vi "SaveReport.vi"(8 "error in (no error)":errorcluster, 9 "Done":bool, 10 "TestResultInformation":T1, 11 "LocalReport in":refnum<class "LocalReport.lvclass">) -> (0 "error out":errorcluster, 3 "LocalReport out":refnum<class "LocalReport.lvclass">)   [LabVIEW 2019, in "LocalReport.lvlib" / "LocalReport.lvclass"]
uses:
  LocalReport.lvclass
  C:/Program Files (x86)/National Instruments/LabVIEW 2019/vi.lib/NI/Event Source Actor/Event Source/Event Source/Event Source.lvclass
  LocalReport.lvclass/LocalReport.ctl
  TestReport.lvclass
  C:/Program Files (x86)/National Instruments/LabVIEW 2019/vi.lib/NI/Event Source Actor/Event Source/Event/Event.lvclass
  <vilib>/NI/Event Source Actor/Event Source/Event/Event.lvclass/Event.ctl
  <vilib>/Utility/file.llb/Write Delimited Spreadsheet (string).vi
  <vilib>/NI/Event Source Actor/Event Source/Event/Event.lvclass
  <vilib>/NI/Event Source Actor/Event Source/Event Source/Event Source.lvclass
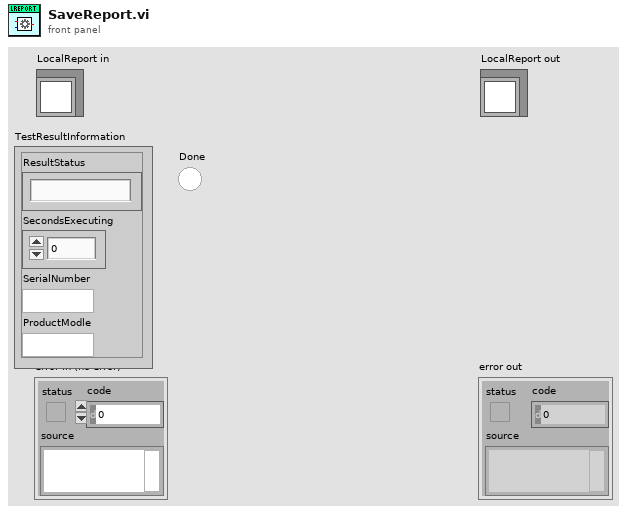
[diagram p1: front panel]
types:
  T1 = cluster{"ResultStatus":string, "SecondsExecuting":dbl, "SerialNumber":string, "ProductModle":string}
  T2 = cluster{"TestResultData":string[][], "SerialNumber":string}[]
  T3 = cluster{"TestResultData":string[][], "SerialNumber":string}
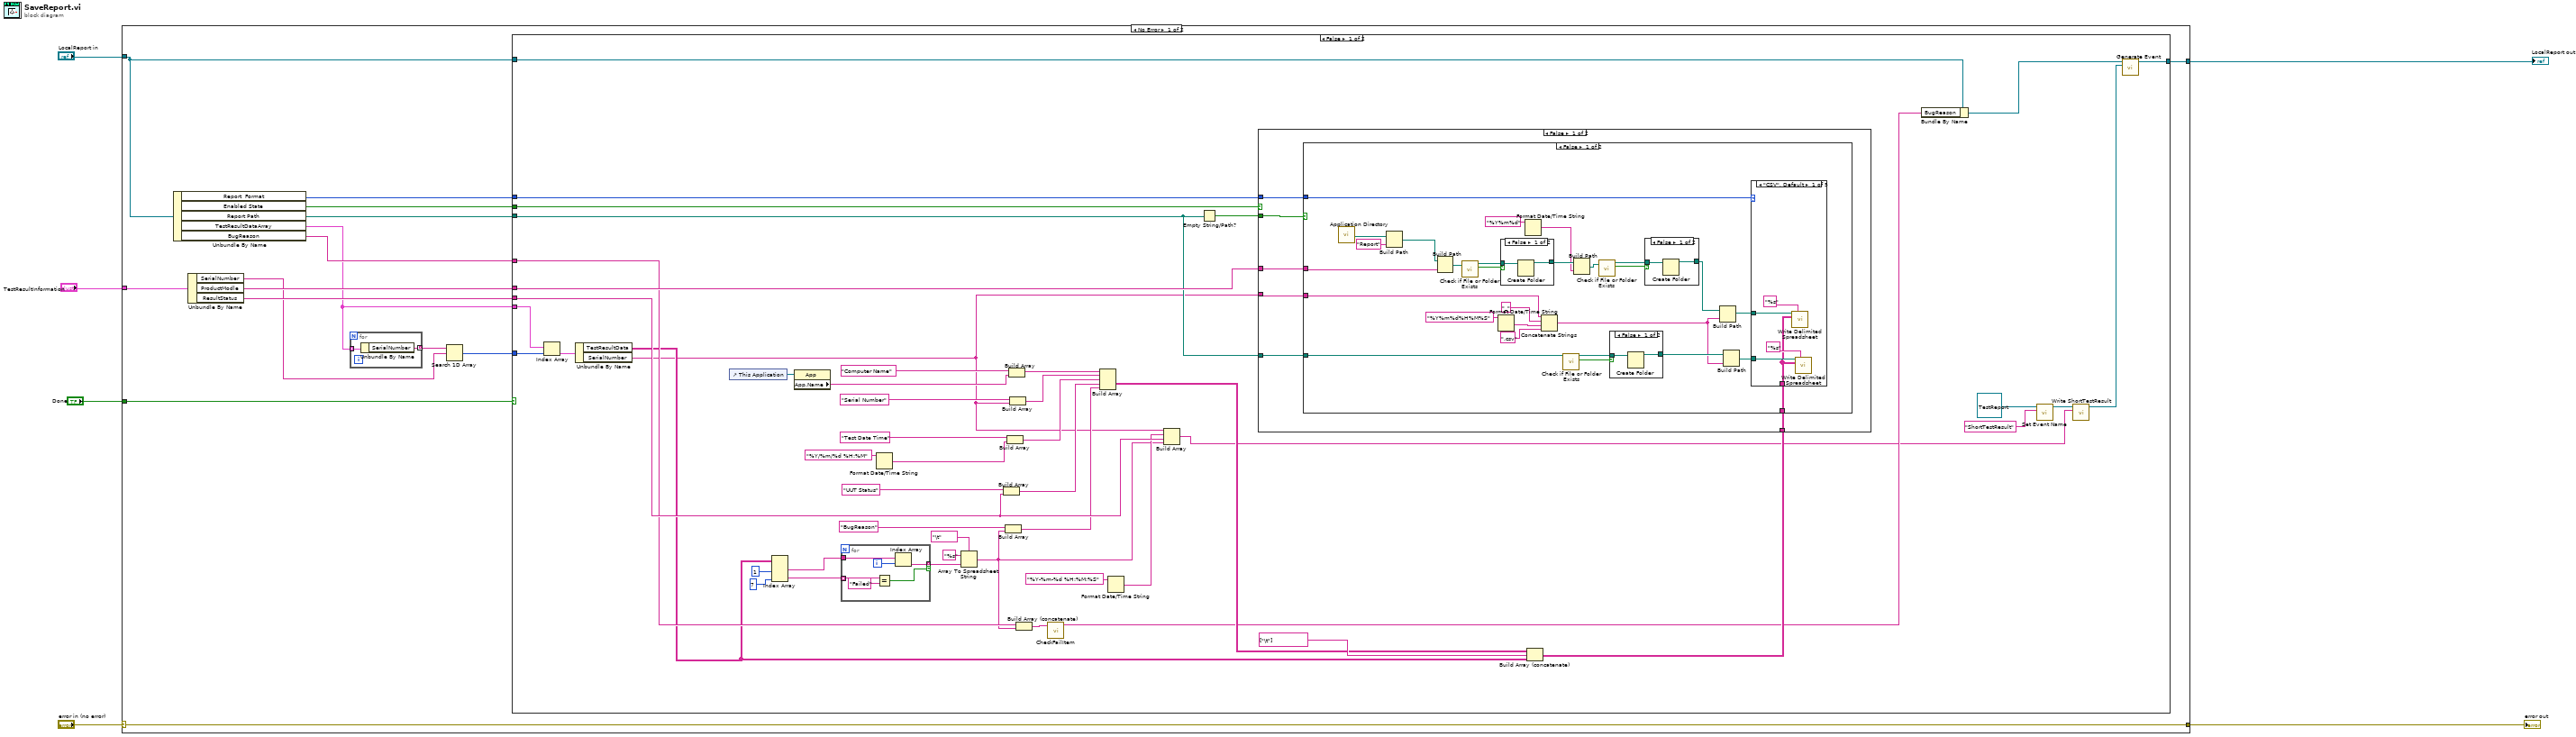
[diagram p0: block diagram]
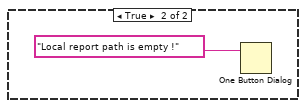
[diagram p9: hidden frame]
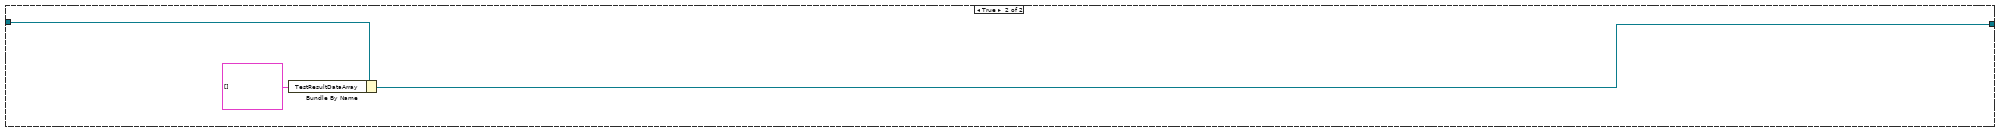
[diagram p11: hidden frame]
diagram:
  n1 = case shown="No Error" "error in (no error)" {
    selector: "error in (no error)" -> [w21 w132]
    tunnel: [w21 w132] -> w5
    tunnel: [w12 w131] -> w3
    tunnel: "LocalReport in" -> [w13 w131]
    tunnel: "TestResultInformation" -> [w20 _]
    tunnel: "Done" -> [w7 _]
    frame No Error {
      n2 = Unbundle By Name(w13) -> ("Report  Format"=w15:enum16{"CSV", "XML", "PDF", "Excel", "TXT"}, "Enabled State"=w16:bool, "Report Path"=w17:path, "TestResultDataArray"=w11:T2, "BugReason"=w14:string[])
      n3 = Unbundle By Name(w20) -> ("SerialNumber"=w9:string, "ProductModle"=w18:string, "ResultStatus"=w19:string)
      n4 = for {
        tunnel: w11 -> [w130] mode=indexing
        tunnel: [w129] -> w10 mode=indexing
        n5 = Unbundle By Name(w130) -> ("SerialNumber"=w129:string)
      }
      n6 = Search 1D Array(1D array=w10, element=w9) -> (index of element=w8:i32)  [unwired: 1 in]
      n7 = case shown="False" w7 {
        tunnel: w19 -> [w70 _]
        tunnel: w18 -> [w69 _]
        tunnel: w17 -> [w68 _]
        tunnel: w16 -> [w67 _]
        tunnel: w15 -> [w66 _]
        tunnel: w14 -> [w65 _]
        tunnel: w13 -> [w64 w128]
        tunnel: [w26 w126] -> w12
        tunnel: w11 -> [w23 _]
        tunnel: w8 -> [w22 _]
        frame False {
          n8 = Index Array(array=w23, index=w22) -> (element=w27:T3)
          n9 = Unbundle By Name(w27) -> ("TestResultData"=w28:string[][], "SerialNumber"=w24:string)
          n10 = control-ref of="This Application"() -> (w41:refnum<vi>)
          n11 = Index Array(array=w28, index (col) #1=1 ("disabled index (col)"), index (col) #2=7 ("disabled index (col)")) -> (element #1=w51:string[], element #2=w53:string[])  [unwired: 2 in]
          n12 = property class="App"(reference=w41) -> ("App.Name"=w40:string)  [unwired: 1 in, 2 out]
          n13 = for {
            tunnel: w53 -> [w125] mode=indexing
            tunnel: [w120] -> w50 mode=indexing if=w123
            tunnel: w51 -> [w121]
            i -> [w122]
            n14 = Equal?(x=w125, y="Failed") -> (x = y?=w123:bool)
            n15 = Index Array(array=w121, index=w122) -> (element=w120:string)
          }
          n16 = Format Date/Time String(time format string (%c)="%Y/%m/%d %H:%M") -> (date/time string=w43:string)  [unwired: 2 in]
          n17 = Array To Spreadsheet String(delimiter (Tab)="\t", array=w50, 3:"%s" ("format string")) -> (spreadsheet string=w25:string)
          n18 = Build Array("UUT Status", w70) -> (w56:string[])
          n19 = Build Array("BugReason", w25) -> (w47:string[])
          n20 = Build Array("Test Date Time", w43) -> (w57:string[])
          n21 = Build Array("Computer Name", w40) -> (w59:string[])
          n22 = Build Array("Serial Number", w24) -> (w58:string[])
          n23 = Build Array (concatenate)(w65, w25) -> (w38:string[])
          n24 = call "CheckFailItem.vi"("in"=w38) -> ("out"=w37:string[])  [unwired: 10 in]
          n25 = Build Array(w59, w58, w57, w56, w47) -> (w45:string[][])
          n26 = Format Date/Time String(time format string (%c)="%Y-%m-%d %H:%M:%S") -> (date/time string=w29:string)  [unwired: 2 in]
          n27 = Build Array(w24, w29, w70, w25) -> (w31:string[])
          n28 = Empty String/Path?(string/path=w68) -> (empty?=w39:bool)
          n29 = Build Array (concatenate)(w45, string[] ["\t"], w28) -> (w42:string[][])
          n30 = case shown="False" w67 {
            tunnel: w42 -> [w76 _]
            tunnel: w69 -> [w75 _]
            tunnel: w68 -> [w74 _]
            tunnel: w24 -> [w73 _]
            tunnel: w39 -> [w72 _]
            tunnel: w66 -> [w71 _]
            frame False {
              n31 = case shown="False" w72 {
                tunnel: w76 -> [w92 _]
                tunnel: w75 -> [w88 _]
                tunnel: w74 -> [w87 _]
                tunnel: w73 -> [w81 _]
                tunnel: w71 -> [w80 _]
                frame False {
                  n32 = call <vilib>:"Application Directory.vi"() -> ("Application Directory"=w79:path)
                  n33 = Build Path(base path=w79, name or relative path="Report") -> (appended path=w78:path)
                  n34 = Build Path(base path=w78, name or relative path=w88) -> (appended path=w103:path)
                  n35 = call <vilib>:"Check if File or Folder Exists.vi"("path"=w103) -> ("file or folder exists?"=w102:bool, "dup path"=w101:path)  [unwired: 8 in, 1 out]
                  n36 = Format Date/Time String(time format string (%c)="%Y%m%d%H%M%S") -> (date/time string=w86:string)  [unwired: 2 in]
                  n37 = case shown="False" w102 {
                    tunnel: w101 -> [w117 w118]
                    tunnel: [w116 w118] -> w100
                    frame False {
                      n38 = Create Folder(path (use dialog)=w117) -> (created path=w116:path)  [unwired: 2 in, 2 out]
                    }
                    frame True {
                    }
                  }
                  n39 = Format Date/Time String(time format string (%c)="%Y%m%d") -> (date/time string=w98:string)  [unwired: 2 in]
                  n40 = Concatenate Strings(w81, "_" ("string"), w86, ".csv" ("name or relative path")) -> (w82:string)
                  n41 = call <vilib>:"Check if File or Folder Exists.vi"("path"=w87) -> ("file or folder exists?"=w90:bool, "dup path"=w91:path)  [unwired: 8 in, 1 out]
                  n42 = Build Path(base path=w100, name or relative path=w98) -> (appended path=w95:path)
                  n43 = call <vilib>:"Check if File or Folder Exists.vi"("path"=w95) -> ("file or folder exists?"=w96:bool, "dup path"=w97:path)  [unwired: 8 in, 1 out]
                  n44 = case shown="False" w90 {
                    tunnel: w91 -> [w111 w112]
                    tunnel: [w110 w112] -> w89
                    frame False {
                      n45 = Create Folder(path (use dialog)=w111) -> (created path=w110:path)  [unwired: 2 in, 2 out]
                    }
                    frame True {
                    }
                  }
                  n46 = case shown="False" w96 {
                    tunnel: w97 -> [w114 w115]
                    tunnel: [w113 w115] -> w94
                    frame False {
                      n47 = Create Folder(path (use dialog)=w114) -> (created path=w113:path)  [unwired: 2 in, 2 out]
                    }
                    frame True {
                    }
                  }
                  n48 = Build Path(base path=w94, name or relative path=w82) -> (appended path=w104:path)
                  n49 = Build Path(base path=w89, name or relative path=w82) -> (appended path=w93:path)
                  n50 = case shown="\"CSV\", Default" w80 {
                    tunnel: w104 -> [w109 _ _ _ _]
                    tunnel: w93 -> [w106 _ _ _ _]
                    tunnel: w92 -> [w105 _ _ _ _]
                    frame "CSV", Default {
                      n51 = call-poly <vilib>:"Write Delimited Spreadsheet.vi"("file path (dialog if empty)"=w109, "format (%s)"="%s", "2D data"=w105) -> ()  [unwired: 11 in, 2 out]
                      n52 = call-poly <vilib>:"Write Delimited Spreadsheet.vi"("file path (dialog if empty)"=w106, "format (%s)"="%s", "2D data"=w105) -> ()  [unwired: 11 in, 2 out]
                    }
                    frame "XML" {
                    }
                    frame "PDF" {
                    }
                    frame "Excel" {
                    }
                    frame "TXT" {
                    }
                  }
                }
                frame True {
                  n53 = One Button Dialog(message="Local report path is empty !") -> ()  [unwired: 1 in, 1 out]
                }
              }
            }
            frame True {
            }
          }
          n54 = Bundle By Name(cluster=w64, "BugReason"=w37) -> (w34:refnum<class "LocalReport.lvclass">)
          n55 = call <vilib>:"Set Event Name.vi"("Name (Generic)"="ShortTestResult", "Event In"=refnum<class "TestReport.lvclass"> refnum ("LocalReport.lvlib:TestReport.lvclass")) -> ("Event Out"=w33:refnum<class "TestReport.lvclass">)  [unwired: 9 in]
          n56 = call-dynamic "Write ShortTestResult.vi"("ShortTestReport"=w31, "TestReport in"=w33) -> ("TestReport out"=w32:refnum<class "TestReport.lvclass">)  [unwired: 8 in, 1 out]
          n57 = call <vilib>:"Generate Event.vi"("Event"=w32, "Event Source In"=w34) -> ("Event Source Out"=w26:refnum<class "LocalReport.lvclass">)  [unwired: 8 in, 1 out]
        }
        frame True {
          n58 = Bundle By Name(cluster=w128, "TestResultDataArray"=T2 []) -> (w126:refnum<class "LocalReport.lvclass">)
        }
      }
    }
    frame Error {
    }
  }
  "error out" <- w5
  "LocalReport out" <- w3
